vi "MPM_Set_Read_Rang_Mode.vi"(8 "error in (no error)":errorcluster, 10 "mode":i32(ring) items=["Manual", "Auto"], 11 ".NET Reference in":refnum<k24>) -> (0 "error out":errorcluster, 3 "Reference out":refnum<k24>)   [LabVIEW 2017]
uses:
  LV_IL_Sample/DLL/InstrumentDLL.dll
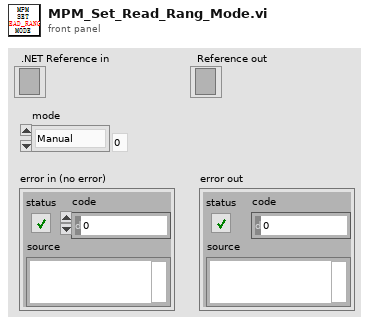
[diagram p1: front panel]
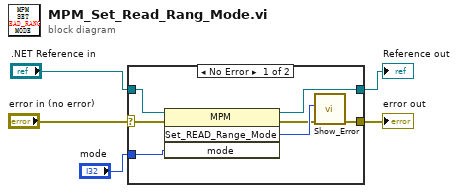
[diagram p0: block diagram]
diagram:
  n1 = case shown="No Error" "error in (no error)" {
    selector: "error in (no error)" -> [w6 w14]
    tunnel: ".NET Reference in" -> [w12 w13]
    tunnel: [w7 w14] -> w4
    tunnel: [w11 w13] -> w3
    tunnel: "mode" -> [w10 _]
    frame No Error {
      n2 = invoke on="调用节点" class="MPM" method="Set_READ_Range_Mode"(reference=w12, error in=w6, "mode"=w10) -> (reference out=w11:refnum<k24>, error out=w8:errorcluster, "Set_READ_Range_Mode"=w9:i32)  [unwired: 1 in, 1 out]
      n3 = call "Show_Error.vi"("error in (no error)"=w8, "Error"=w9) -> ("error out"=w7:errorcluster)  [unwired: 9 in]
    }
    frame Error {
    }
  }
  "Reference out" <- w3
  "error out" <- w4
